vi "Range_To_List.vi"(11 "Range String":string) -> (2 "Array":i32[](array[numeric]), 3 "List":string)   [LabVIEW 2021]
doc: "Converts string containing range to a list"
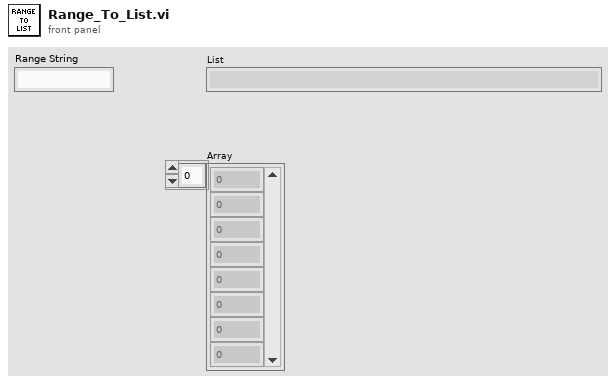
[diagram p1: front panel]
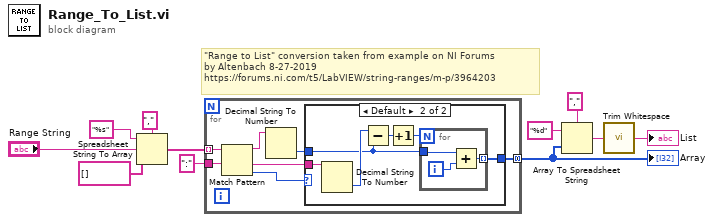
[diagram p0: block diagram]
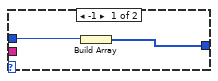
[diagram p2: hidden frame]
diagram:
  # "\"Range to List\" conversion taken from example on NI Forums\nby Altenbach 8-27-2019\nhttps://forums.ni.com/t5/LabVIEW/string-ranges/m-p/3964203"
  n1 = Spreadsheet String To Array(delimiter (Tab)=",", format string="%s", spreadsheet string="Range String", array type (2D Dbl)=string[] []) -> (array=w3:string[])
  n2 = for {
    tunnel: w3 -> [w18] mode=indexing
    tunnel: ":" ("regular expression") -> [w14]
    tunnel: [w13] -> w6 mode=concatenating
    n3 = Match Pattern(string=w18, regular expression=w14) -> (before substring=w15:string, after substring=w16:string, offset past match=w17:i32)  [unwired: 1 in, 1 out]
    n4 = Decimal String To Number(string=w15) -> (number=w12:i32)  [unwired: 2 in, 1 out]
    n5 = case shown="Default" w17 {
      tunnel: w16 -> [_ w26]
      tunnel: [w19 w22] -> w13
      tunnel: w12 -> [w20 w21]
      frame -1 {
        n6 = Build Array(w20) -> (w19:i32[])
      }
      frame Default {
        n7 = Decimal String To Number(string=w26) -> (number=w25:i32)  [unwired: 2 in, 1 out]
        n8 = Subtract(x=w25, y=w21) -> (x-y=w24:i32)
        n9 = Increment(x=w24) -> (x+1=w23:i32)
        n10 = for {
          N: w23 -> [_]
          tunnel: [w28] -> w22 mode=indexing
          tunnel: w21 -> [w27]
          i -> [w29]
          n11 = Add(x=w27, y=w29) -> (x+y=w28:i32)
        }
      }
    }
  }
  "Array" <- w6
  n12 = Array To Spreadsheet String(delimiter (Tab)=",", array=w6, 3:"%d" ("format string")) -> (spreadsheet string=w9:string)
  n13 = call <vilib>:"Trim Whitespace.vi"("string"=w9) -> ("trimmed string"=→"List":string)  [unwired: 1 in]
